vi "Wait_PTB.vi"(0 "Data Task in":refnum<k21>, 5 "data task error in":errorcluster, 7 "#DAQ outputs (1-13)":i32, 9 "PS VISA in":refnum<visa-resource-name>, 11 "PS error in":errorcluster caption="PS error in (no error)", 12 "Wait Filepath":path=path "C:/Users/ga11/Desktop/VI/results/3PtestChrgRest.lvm" caption="Filename", 13 "Wait time":dbl) -> (4 "data task out":refnum<k21>, 6 "data task error out":errorcluster, 10 "PS Visa Out":refnum<visa-resource-name>, 15 "PS error out":errorcluster)   [LabVIEW 2020]
uses:
  Drivers-Essentials/NH Research Regenerative Test Series.lvlib
  Parallel-Current-Analysis-Platform-PCAP/parallel_testbed/IT-M3400-LV/IT-M3400/IT-M3400.lvlib
panel:
  out "Ave Current (A)":dbl
  out "Ave Voltage (V)":dbl
  out "WaitElapsed Time (s)":i32 caption="Elapsed Time (s)"
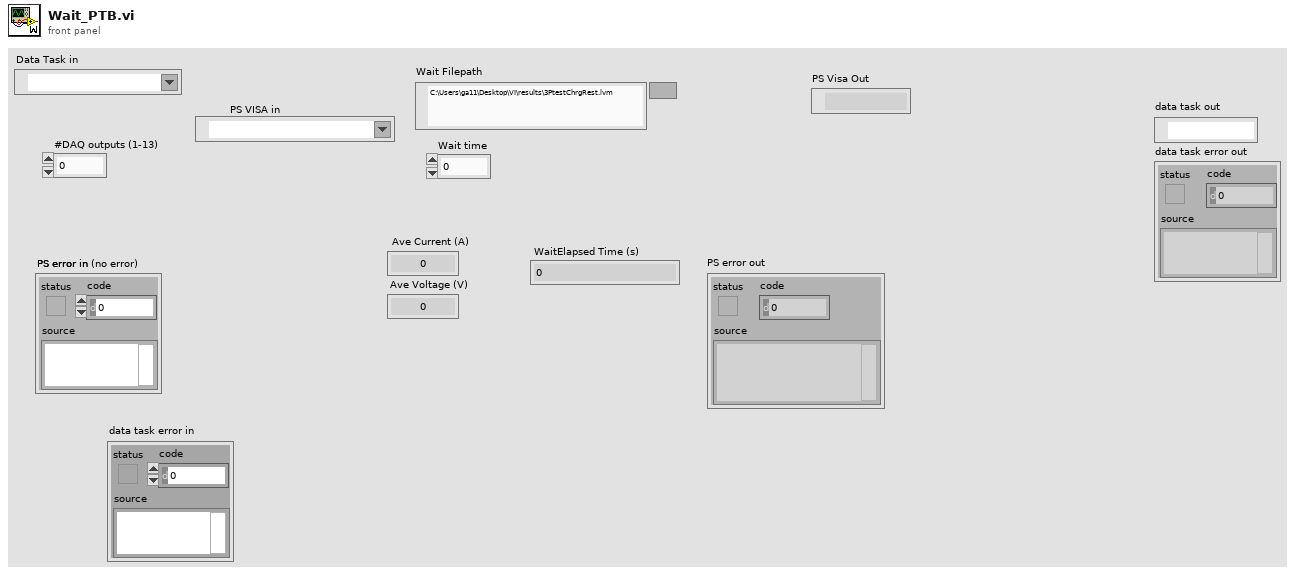
[diagram p1: front panel]
types:
  T1 = cluster{"Voltage Enabled":bool, "Current Enabled":bool, "Power Enabled":bool, "Resistance Enabled":bool}
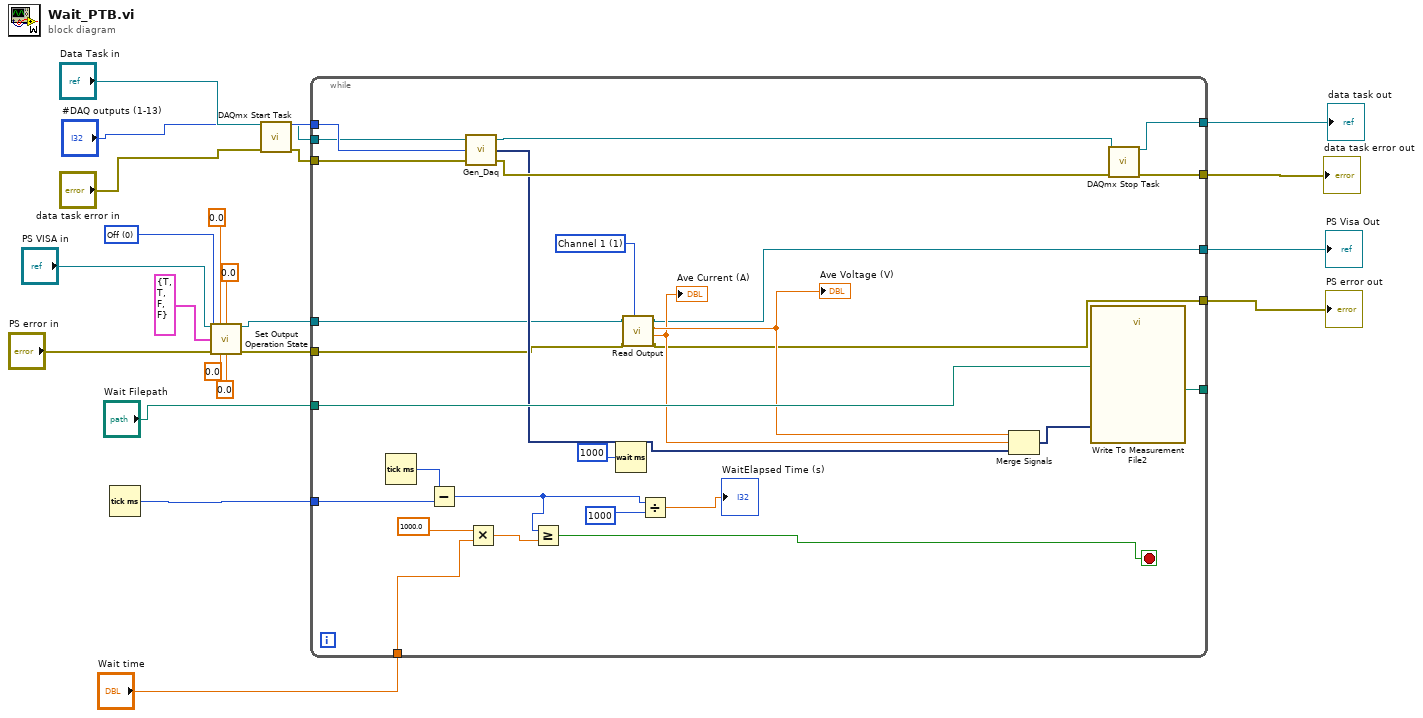
[diagram p0: block diagram]
diagram:
  w8 = 0 items=["Off", "Standby", "Charge", "Discharge", "Battery"] ("Mode (0: Off)")
  n1 = Tick Count (ms)() -> (millisecond timer value=w21:u32)
  n2 = call "Set Output Operation State.vi"("VISA resource name"="PS VISA in", "Voltage Setpoint (0 V)"=0.0, "Current Setpoint (0 A)"=0.0, "Mode (0: Off)"=w8, "Enable"=T1 {"Voltage Enabled"=TRUE, "Current Enabled"=TRUE, "Power Enabled"=FALSE, "Resistance Enabled"=FALSE}, "error in (no error)"="PS error in", "Power Setpoint (0 W)"=0.0, "Resistance Setpoint (0 Ohms)"=0.0) -> ("VISA resource name out"=w9:refnum<visa-resource-name>, "error out"=w5:errorcluster)  [unwired: 6 in]
  n3 = call <vilib>:"DAQmx Start Task.vi"("task/channels in"="Data Task in", "error in"="data task error in") -> ("task out"=w12:refnum<k21>, "error out"=w11:errorcluster)  [unwired: 12 in]
  n4 = while {
    tunnel: "Wait time" -> [w47]
    tunnel: [w44] -> _
    tunnel: w21 -> [w43]
    tunnel: "Wait Filepath" -> [w42]
    tunnel: [w25] -> w19
    tunnel: [w24] -> w18
    tunnel: "#DAQ outputs (1-13)" -> [w36]
    tunnel: w12 -> [w35]
    tunnel: w11 -> [w34]
    tunnel: [w33] -> w14
    tunnel: [w32] -> w13
    tunnel: w9 -> [w29]
    tunnel: w5 -> [w28]
    stop <- w48 stop-if-true
    w23 = 1 items=["Channel 1"=1, "Channel 2"=2, "Channel 3"=3, "Channel 4"=4, "Channel 5"=5, "Channel 6"=6, "Channel 7"=7, "Channel 8"=8, "Channel 8"=9, "Channel 10"=10, "Channel 11"=11, "Channel 12"=12, "Channel 13"=13, "Channel 14"=14, "Channel 15"=15, "Channel 16"=16] ("Channel")
    n5 = Tick Count (ms)() -> (millisecond timer value=w49:u32)
    n6 = Subtract(x=w49, y=w43) -> (x-y=w30:u32)
    n7 = call "Gen_Daq.vi"("error in"=w34, "#DAQ outputs (1-13)"=w36, "task/channels in"=w35) -> ("error out"=w37:errorcluster, "DaQ_output"=w31:dynamicdata, "task out"=w38:refnum<k21>)
    n8 = Multiply(x=1000.0, y=w47) -> (x*y=w45:dbl)
    n9 = Greater Or Equal?(x=w30, y=w45) -> (x >= y?=w48:bool)
    n10 = Wait (ms)(milliseconds to wait=1000) -> ()  [unwired: 1 out]
    n11 = call "Read Output.vi"("Channel"=w23, "error in"=w28, "VISA resource name"=w29) -> ("error out"=w24:errorcluster, "Actual Current Level (A)"=w26:dbl, "Actual Voltage Level (V)"=w27:dbl, "VISA resource name out"=w25:refnum<visa-resource-name>)  [unwired: 5 in]
    "Ave Current (A)" <- w26
    "Ave Voltage (V)" <- w27
    n12 = Divide(x=w30, y=1000) -> (x/y=→"WaitElapsed Time (s)":dbl)
    n13 = Merge Signals "Merge Signals"(w27, w26, w31) -> (w39:dynamicdata)
    n14 = call "Write To Measurement File2"("Signals"=w39, "Filename"=w42) -> ("Filename Out"=w44:path)  [unwired: 15 in, 2 out]
    n15 = call <vilib>:"DAQmx Stop Task.vi"("task/channels in"=w38, "error in"=w37) -> ("task out"=w33:refnum<k21>, "error out"=w32:errorcluster)  [unwired: 12 in]
  }
  "PS Visa Out" <- w19
  "PS error out" <- w18
  "data task out" <- w14
  "data task error out" <- w13
